vi "CAN Name validate.vi"(8 "error in":errorcluster caption="error out", 11 "Gas Name in":T1) -> (0 "error out":errorcluster, 2 "found Unit out":T1, 3 "valid Name out":T1)   [LabVIEW 2020, in "CAN Konfig.lvlib"]
uses:
  CAN Konfig.lvlib
  Visualisierungs Elemente/String - Ausgabefeld.ctl
  <vilib>/regexp/Match Regular Expression.xnode
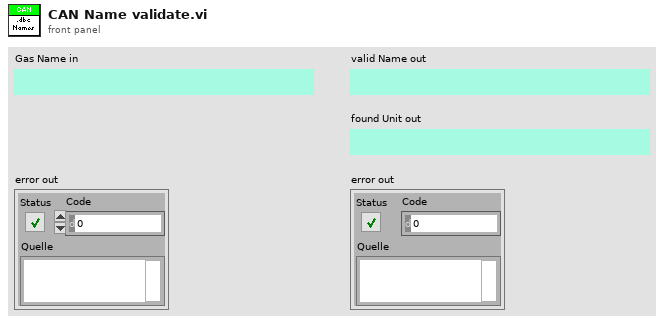
[diagram p1: front panel]
types:
  T1 = typedef "String - Ausgabefeld.ctl" = string
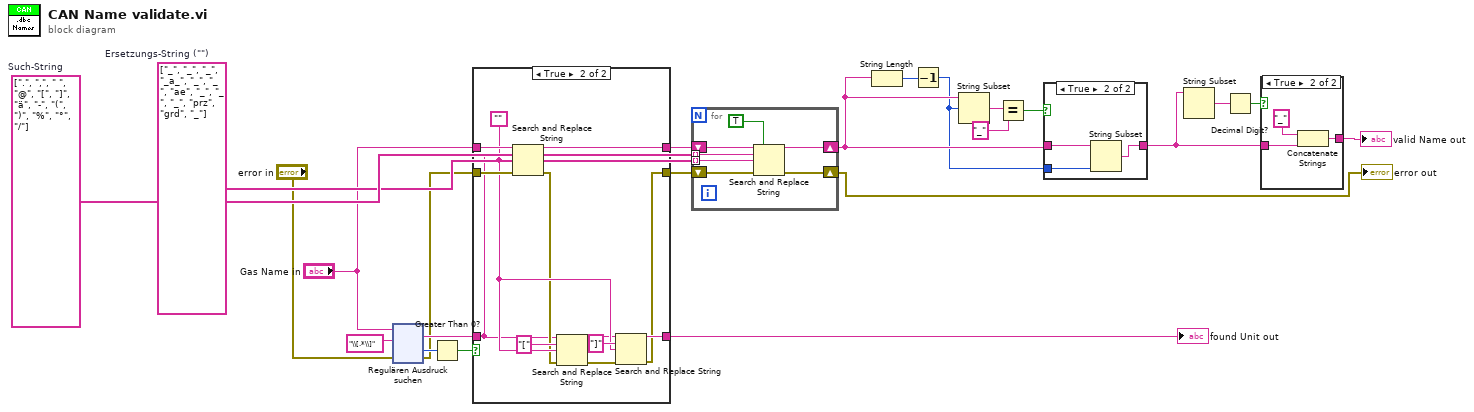
[diagram p0: block diagram]
diagram:
  w18 = string[] ["_", "_", "_", "_a_", "_", "_", "ae", "_", "_", "_", "prz", "grd", "_"]  # Ersetzungs-String ("")
  w19 = string[] [".", ",", " ", "@", "[", "]", "ä", "-", "(", ")", "%", "°", "/"]  # Such-String
  n1 = xnode "Regulären Ausdruck suchen"("Eingangs-String"="Gas Name in", "Regulärer Ausdruck"="\\[.*\\]", "Fehler (Eingang)"="error in") -> ("Komplette Übereinstimmung"=w21:string, "Offset nach Übereinstimmung"=w17:i32, "Fehler (Ausgang)"=w14:errorcluster)  [unwired: 3 in, 2 out]
  n2 = Greater Than 0?(x=w17) -> (x > 0?=w22:bool)
  n3 = case shown="True" w22 {
    tunnel: w21 -> [_ w27]
    tunnel: [_ w34] -> w20
    tunnel: "Gas Name in" -> [w25 w37]
    tunnel: [w25 w36] -> w12
    tunnel: w14 -> [w24 w35]
    tunnel: [w24 w28] -> w13
    frame False {
    }
    frame True {
      w30 = ""
      n4 = Search and Replace String(input string=w37, search string=w27, replace string=w30, error in=w35) -> (result string=w36:string, error out=w29:errorcluster)  [unwired: 4 in, 2 out]
      n5 = Search and Replace String(input string=w27, search string="[" ("Such-String"), replace string=w30, error in=w29) -> (result string=w26:string, error out=w33:errorcluster)  [unwired: 4 in, 2 out]
      n6 = Search and Replace String(input string=w26, search string="]" ("Such-String"), replace string=w30, error in=w33) -> (result string=w34:string, error out=w28:errorcluster)  [unwired: 4 in, 2 out]
    }
  }
  "found Unit out" <- w20
  n7 = for {
    tunnel: w19 -> [w43] mode=indexing
    tunnel: w18 -> [w42] mode=indexing
    shift-right: [w41] -> w9
    shift-left: w12 -> [w44]
    shift-right: [w39] -> w1
    shift-left: w13 -> [w38]
    n8 = Search and Replace String(replace all?=TRUE ("Alle ersetzen? (F)"), input string=w44, search string=w43, replace string=w42, error in=w38) -> (result string=w41:string, error out=w39:errorcluster)  [unwired: 3 in, 2 out]
  }
  "error out" <- w1
  n9 = String Length(string=w9) -> (length=w8:i32)
  n10 = Decrement(x=w8) -> (x-1=w6:i32)
  n11 = String Subset(string=w9, offset (0)=w6) -> (substring=w11:T1)  [unwired: 1 in]
  n12 = Equal?(x=w11, y=T1 "_") -> (x = y?=w10:bool)
  n13 = case shown="True" w10 {
    tunnel: w9 -> [w45 w48]
    tunnel: [w45 w47] -> w3
    tunnel: w6 -> [_ w46]
    frame False {
    }
    frame True {
      n14 = String Subset(string=w48, length (rest)=w46) -> (substring=w47:T1)  [unwired: 1 in]
    }
  }
  n15 = String Subset(string=w3) -> (substring=w5:T1)  [unwired: 2 in]
  n16 = Decimal Digit?(1:w5) -> (0:w4:bool)
  n17 = case shown="True" w4 {
    tunnel: w3 -> [w49 w52]
    tunnel: [w49 w50] -> w2
    frame False {
    }
    frame True {
      n18 = Concatenate Strings(T1 "_" ("String"), w52) -> (w50:string)
    }
  }
  "valid Name out" <- w2
